vi "Get Current State.vi"(8 "error in":errorcluster, 11 "History":refnum<class "History.lvclass">) -> (0 "error out":errorcluster, 2 "Current State":string, 4 "Add Undo":bool)   [LabVIEW 2020, in "lv_icon.lvlib" / "History.lvlib" / "History.lvclass"]
doc: "Gets the state the history buffer was last set to as well as if the Add Undo flag was set."
uses:
  History.lvclass
  History.lvclass/History.ctl
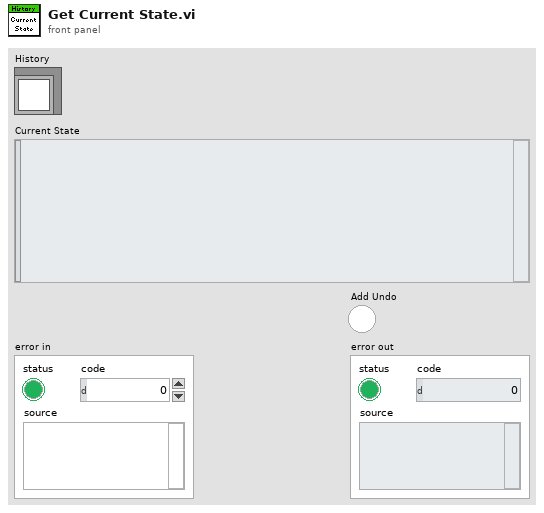
[diagram p1: front panel]
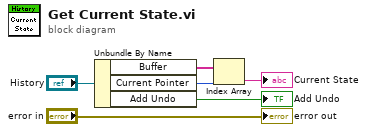
[diagram p0: block diagram]
diagram:
  n1 = Unbundle By Name("History") -> ("Buffer"=w4:string[], "Current Pointer"=w3:i32, "Add Undo"=→"Add Undo":bool)
  n2 = Index Array(array=w4, index=w3) -> (element=→"Current State":string)
  "error out" <- "error in"
